vi "Acquisition Message Loop.vi"(6 "Acquisition Status Notifier":refnum<notifier>, 8 "error in (no error)":errorcluster, 9 "Data Queue":refnum<queue>, 10 "Data Notifier":refnum<notifier>, 11 "Message Queues":T1) -> (0 "error out":errorcluster)   [LabVIEW 2021, in "Acquisition.lvlib"]
doc: "Message loop for handling messages pertaining to the acquisition of data from the hardware."
uses:
  Acquisition.lvlib
  support/Message Queue/All Message Queues.ctl
  support/Message Queue/Message Cluster.ctl
  Acquired Data.ctl
  controls/Acquisition Status.ctl
  Acquisition State.ctl
  support/Message Queue/Enqueue Message (Single).vi
  <vilib>/Utility/error.llb/Error Cluster From Error Code.vi
  <vilib>/ErrorRing/Error Ring.xnode
  support/Message Queue/Message Queue.lvlib
panel:
  out "msgctr":i32
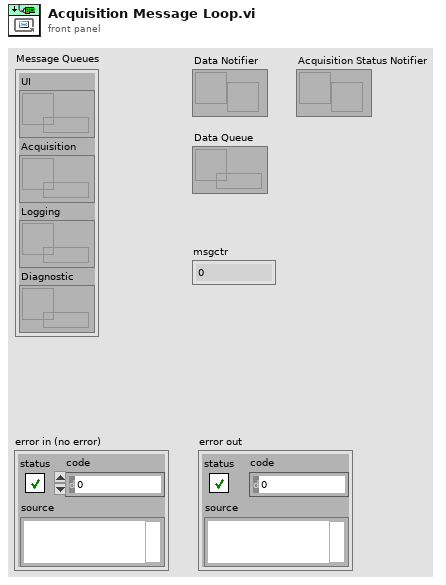
[diagram p1: front panel]
types:
  T1 = typedef "Message Queue.lvlib/All Message Queues.ctl" = cluster{"UI":refnum<queue>, "Acquisition":refnum<queue>, "Logging":refnum<queue>, "Diagnostic":refnum<queue>}
  T2 = typedef "Acquisition.lvlib/Acquisition State.ctl" = enum16{"Idle", "Acquiring"}
  T3 = typedef "Acquisition.lvlib/Host Resources.ctl" = cluster{"NI Software":T4[], "IO Devices":T5[]}
  T4 = typedef "Acquisition.lvlib/Host Software Package.ctl" = cluster{"ID":string, "Version":string}
  T5 = typedef "Acquisition.lvlib/Host IO Resource.ctl" = cluster{"Model Number":u32, "Alias":string, "Product Name":string, "Is Device":bool, "Is Chassis":bool, "Is Simulated":bool, "Slot":i32}
  T6 = typedef "Acquisition.lvlib/Hardware Configuration.ctl" = cluster{"Channel Settings":T7[], "Sensor Intervals":T10[], "Sensor Token":T12, "IO Context":T13}
  T7 = typedef "Acquisition.lvlib/Channel Settings.ctl" = cluster{"Name":string, "Terminal Information":cluster{"IO Device":T8, "Channel":i32, "Sensor Type":T9}, "Calibration Information":cluster{"Excitation Voltage":dbl, "Calibration Factor":dbl, "Zero Value":dbl, "Calibration Formula":string, "Units":string}}
  T8 = typedef "Acquisition.lvlib/IO Device.ctl" = enum16{"none", "9219", "9401"}
  T9 = typedef "Acquisition.lvlib/Sensor Type.ctl" = enum16{"Voltage", "Load", "Pressure", "Encoder"}
  T10 = typedef "Interval Timer.lvlib/Repeat Interval.ctl" = cluster{"Interval":T11, "Count":i32}
  T11 = typedef "Interval Timer.lvlib/Interval Length.ctl" = enum16{"Manual control", "1 second", "10 seconds", "30 seconds", "60 seconds", "600 seconds", "1200 seconds", "3600 seconds"}
  T12 = typedef "Interval Timer.lvlib/Interval Token.ctl" = cluster{"Next reading in ms":u32, "Interval Index":i32, "Interval Occurrence":i32}
  T13 = typedef "Acquisition.lvlib/IO Context.ctl" = cluster{"API":T14, "API Wire":variant}
  T14 = typedef "Acquisition.lvlib/IO API.ctl" = enum16{"Simulated", "DAQmx"}
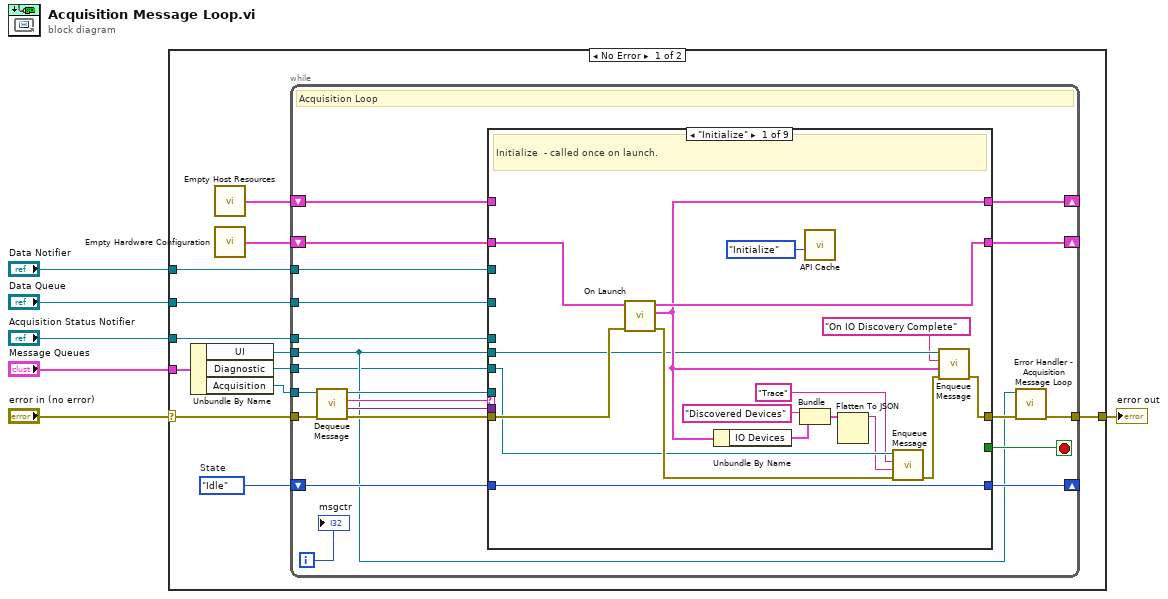
[diagram p0: block diagram]
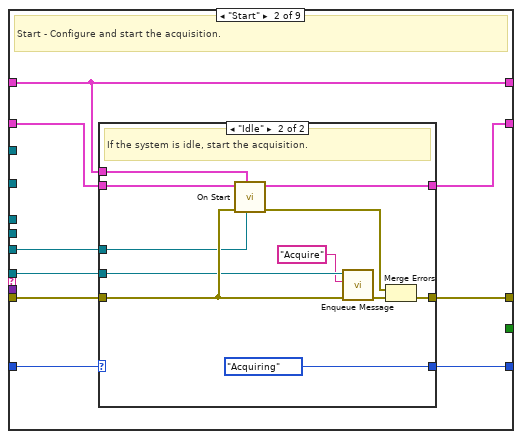
[diagram p2: hidden frame]
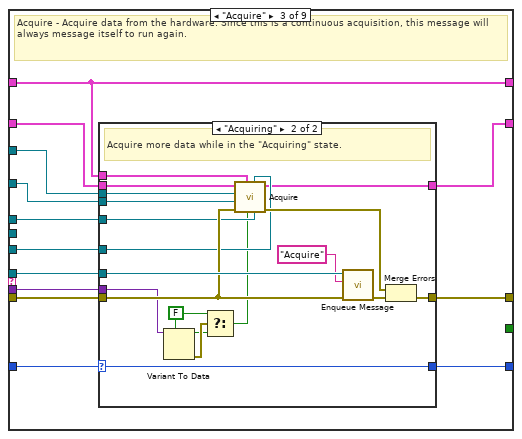
[diagram p4: hidden frame]
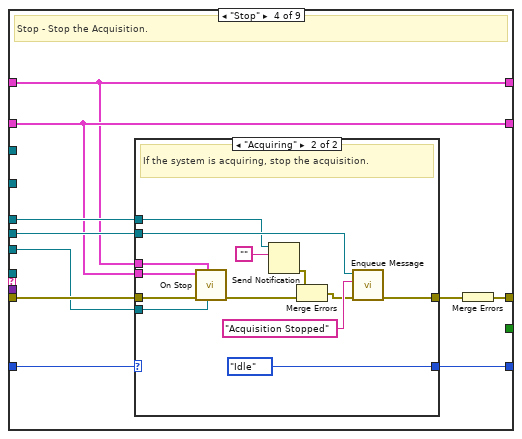
[diagram p6: hidden frame]
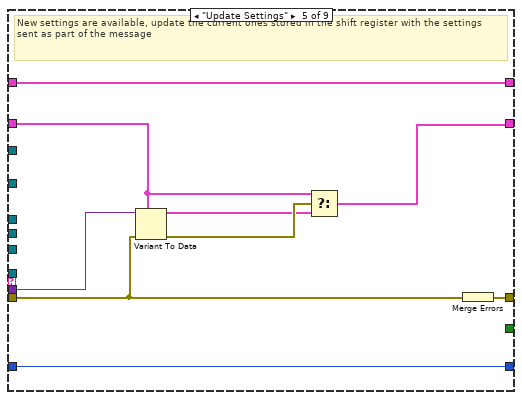
[diagram p8: hidden frame]
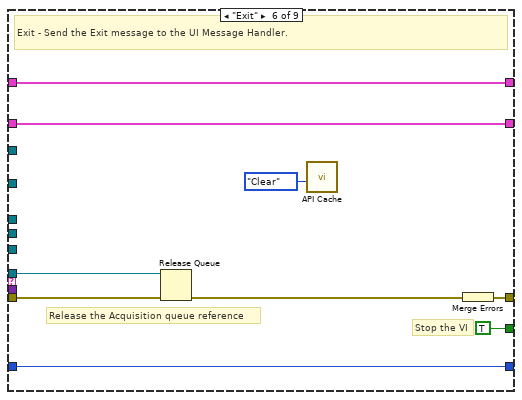
[diagram p9: hidden frame]
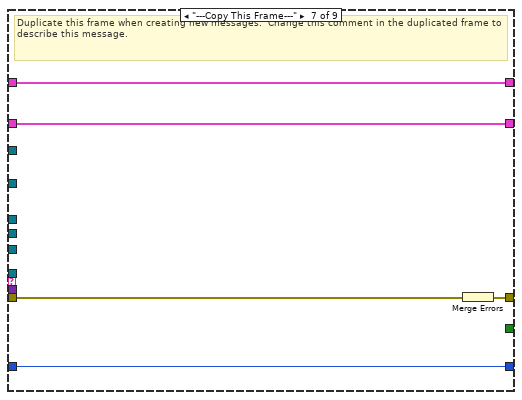
[diagram p10: hidden frame]
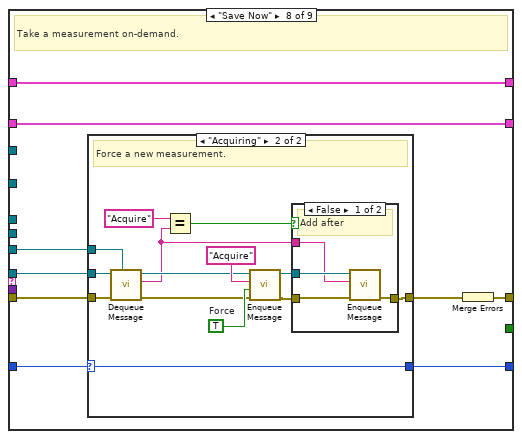
[diagram p11: hidden frame]
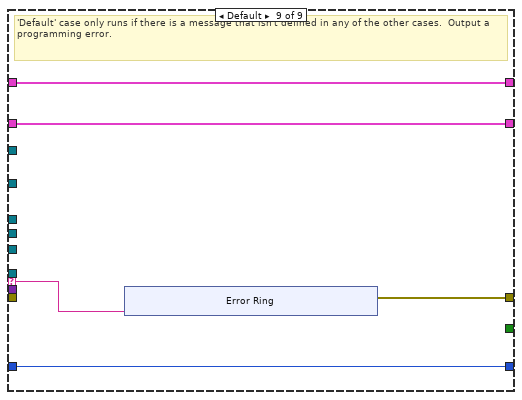
[diagram p14: hidden frame]
diagram:
  n1 = case shown="No Error" "error in (no error)" {
    selector: "error in (no error)" -> [w15 w205]
    tunnel: "Message Queues" -> [w18 _]
    tunnel: [w16 w205] -> w5
    tunnel: "Data Notifier" -> [w13 _]
    tunnel: "Data Queue" -> [w12 _]
    tunnel: "Acquisition Status Notifier" -> [w9 _]
    frame No Error {
      w11 = Acquisition_State."Idle"  # State
      n2 = Unbundle By Name(w18) -> ("UI"=w14:refnum<queue>, "Diagnostic"=w10:refnum<queue>, "Acquisition"=w17:refnum<queue>)
      n3 = call "Empty Host Resources.vi"() -> ("Host Resources"=w7:T3)
      n4 = call "Empty Hardware Configuration.vi"() -> ("Hardware Configuration"=w8:T6)
      n5 = while {
        tunnel: w17 -> [w32]
        shift-right: [w38] -> _
        shift-left: w8 -> [w39]
        tunnel: w14 -> [w24]
        tunnel: w13 -> [w31]
        tunnel: w12 -> [w30]
        shift-right: [w28] -> _
        shift-left: w11 -> [w29]
        tunnel: w15 -> [w36]
        tunnel: [w27] -> w16
        tunnel: w10 -> [w22]
        tunnel: w9 -> [w21]
        shift-right: [w19] -> _
        shift-left: w7 -> [w20]
        i -> [w23]
        stop <- w37 stop-if-true
        # "Acquisition Loop"
        n6 = call "Dequeue Message.vi"("error in (no error)"=w36, "Message Queue"=w32) -> ("error out"=w35:errorcluster, "Message Data"=w33:variant, "Message"=w34:string, "dup Message Queue"=w25:refnum<queue>)  [unwired: 6 in]
        n7 = case "Message Cases" shown="\"Initialize\"" w34 {
          selector: w34 -> [_ _ _ _ _ _ _ _ w194]
          tunnel: w25 -> [_ w63 w91 _ _ w152 _ w166 _]
          tunnel: w35 -> [w53 w64 w90 w123 w144 w154 w162 w168 _]
          tunnel: [w52 w65 w92 w124 w148 w156 w160 w171 w195] -> w26
          tunnel: w39 -> [w55 w60 w83 w117 w141 w155 w161 w165 w197]
          tunnel: [w54 w59 w82 w117 w140 w155 w161 w165 w197] -> w38
          tunnel: [_ _ _ _ _ TRUE _ _ _] -> w37
          tunnel: w33 -> [_ _ w85 _ w147 _ _ _ _]
          tunnel: w24 -> [w47 _ _ w119 _ _ _ _ _]
          tunnel: w31 -> [_ _ w89 _ _ _ _ _ _]
          tunnel: w30 -> [_ _ w88 _ _ _ _ _ _]
          tunnel: w29 -> [w56 w61 w86 w121 w143 w151 w159 w170 w196]
          tunnel: [w56 w62 w87 w120 w143 w151 w159 w169 w196] -> w28
          tunnel: w22 -> [w48 w57 w81 w116 _ _ _ w164 _]
          tunnel: w21 -> [_ _ w84 w118 _ _ _ _ _]
          tunnel: w20 -> [_ w58 w80 w115 w142 w150 w158 w163 w193]
          tunnel: [w51 w58 w80 w115 w142 w150 w158 w163 w193] -> w19
          frame "Initialize" {
            # "Initialize  - called once on launch."
            n8 = call "On Launch.vi"("error in (no error)"=w53, "Hardware Resources in"=w55) -> ("error out"=w50:errorcluster, "Host Resources"=w51:T3, "Hardware Resources out"=w54:T6)  [unwired: 7 in]
            n9 = Unbundle By Name(w51) -> ("IO Devices"=w44:T5[])
            n10 = Bundle("Message"="Discovered Devices", "IO Devices"=w44) -> (w42:cluster{"Message":string, "IO Devices":T5[]})  [unwired: 1 in]
            n11 = call "API Cache.vi"("Action"=enum16{"Initialize", "Get or Open", "Clear"}."Initialize") -> ()  [unwired: 9 in, 2 out]
            n12 = Flatten To JSON(anything=w42) -> (JSON string=w41:string)  [unwired: 2 in, 1 out]
            n13 = call-poly "Enqueue Message.vi"("error in (no error)"=w50, "Message Data"=w41, "Message"="Trace", "Message Queue"=w48) -> ("error out"=w49:errorcluster)  [unwired: 6 in, 1 out]
            n14 = call-poly "Enqueue Message.vi"("error in (no error)"=w49, "Message Data"=w51, "Message"="On IO Discovery Complete", "Message Queue"=w47) -> ("error out"=w52:errorcluster)  [unwired: 6 in, 1 out]
          }
          frame "Start" {
            # "Start - Configure and start the acquisition."
            n15 = case shown="\"Idle\"" w61 {
              selector: w61 -> [w66 _]
              tunnel: [w67 w79] -> w65
              tunnel: w60 -> [w68 w78]
              tunnel: w64 -> [w67 w77]
              tunnel: w63 -> [_ w75]
              tunnel: [w68 w71] -> w59
              tunnel: [w66 Acquisition_State."Acquiring" ("Acquisition State")] -> w62
              tunnel: w58 -> [_ w70]
              tunnel: w57 -> [_ w69]
              frame "Acquiring" {
                # "The system is already acquiring. Ignore the \"Start\" message."
              }
              frame "Idle" {
                # "If the system is idle, start the acquisition."
                n16 = call "On Start.vi"("Diagnostics Queue"=w69, "Host Resources"=w70, "error in (no error)"=w77, "Hardware Configuration in"=w78) -> ("error out"=w72:errorcluster, "Hardware Configuration out"=w71:T6)  [unwired: 6 in]
                n17 = call-poly "Enqueue Message.vi"("error in (no error)"=w77, "Message"="Acquire", "Message Queue"=w75) -> ("error out"=w76:errorcluster)  [unwired: 7 in, 1 out]
                n18 = Merge Errors(w72, w76) -> (w79:errorcluster)
              }
            }
          }
          frame "Acquire" {
            # "Acquire - Acquire data from the hardware. Since this is a continuous acquisition, this message will always message itself to run again."
            n19 = case shown="\"Acquiring\"" w86 {
              selector: w86 -> [w93 w106]
              tunnel: [w94 w114] -> w92
              tunnel: w91 -> [_ w112]
              tunnel: w90 -> [w94 w105]
              tunnel: [w95 w97] -> w82
              tunnel: w83 -> [w95 w110]
              tunnel: w89 -> [_ w108]
              tunnel: w88 -> [_ w107]
              tunnel: [w93 w106] -> w87
              tunnel: w85 -> [_ w104]
              tunnel: w84 -> [_ w100]
              tunnel: w81 -> [_ w99]
              tunnel: w80 -> [_ w98]
              frame "Idle" {
                # "Ignore \"Acquire\" messages when the acquisition is idle."
              }
              frame "Acquiring" {
                w103 = FALSE
                # "Acquire more data while in the \"Acquiring\" state."
                n20 = Variant To Data(type=w103, Variant=w104) -> (data=w101:bool, error out=w102:errorcluster)  [unwired: 1 in]
                n21 = Select(t=w103, s=w102, f=w101) -> (s? t:f=w96:bool)
                n22 = call "Acquire.vi"("Acquisition Status Notifier"=w100, "Diagnostics Queue"=w99, "Force?"=w96, "Host Resources"=w98, "error in (no error)"=w105, "Data Queue"=w107, "Data Notifier"=w108, "Hardware Resources in"=w110) -> ("error out"=w111:errorcluster, "Hardware Resources out"=w97:T6)  [unwired: 2 in]
                n23 = call-poly "Enqueue Message.vi"("error in (no error)"=w105, "Message"="Acquire", "Message Queue"=w112) -> ("error out"=w113:errorcluster)  [unwired: 7 in, 1 out]
                n24 = Merge Errors(w111, w113) -> (w114:errorcluster)
              }
            }
          }
          frame "Stop" {
            # "Stop - Stop the Acquisition."
            n25 = case shown="\"Acquiring\"" w121 {
              selector: w121 -> [w125 _]
              tunnel: w123 -> [w126 w139]
              tunnel: [w126 w135] -> w122
              tunnel: w117 -> [_ w137]
              tunnel: [w125 Acquisition_State."Idle" ("State")] -> w120
              tunnel: w119 -> [_ w134]
              tunnel: w118 -> [_ w130]
              tunnel: w116 -> [_ w128]
              tunnel: w115 -> [_ w127]
              frame "Idle" {
                # "The system is already idle. Ignore the \"Stop\" message."
              }
              frame "Acquiring" {
                # "If the system is acquiring, stop the acquisition."
                n26 = call "On Stop.vi"("Diagnostics Queue"=w128, "Host Resources"=w127, "error in (no error)"=w139, "Hardware Resources in"=w137) -> ("error out"=w138:errorcluster)  [unwired: 6 in, 1 out]
                n27 = Send Notification(notification="", notifier=w130) -> (error out=w131:errorcluster)  [unwired: 1 in, 1 out]
                n28 = Merge Errors(w131, w138) -> (w132:errorcluster)
                n29 = call-poly "Enqueue Message.vi"("error in (no error)"=w132, "Message"="Acquisition Stopped", "Message Queue"=w134) -> ("error out"=w135:errorcluster)  [unwired: 7 in, 1 out]
              }
            }
            n30 = Merge Errors(w122) -> (w124:errorcluster)
          }
          frame "Update Settings" {
            # "New settings are available, update the current ones stored in the shift register with the settings sent as part of the message"
            n31 = Variant To Data(error in=w144, type=w141, Variant=w147) -> (data=w145:T6, error out=w146:errorcluster)
            n32 = Select(t=w141, s=w146, f=w145) -> (s? t:f=w140:T6)
            n33 = Merge Errors(w144) -> (w148:errorcluster)
          }
          frame "Exit" {
            # "Release the Acquisition queue reference"
            # "Stop the VI"
            # "Exit - Send the Exit message to the UI Message Handler."
            n34 = Release Queue(queue=w152, error in (no error)=w154) -> (error out=w153:errorcluster)  [unwired: 1 in, 2 out]
            n35 = call "API Cache.vi"("Action"=enum16{"Initialize", "Get or Open", "Clear"}."Clear") -> ()  [unwired: 9 in, 2 out]
            n36 = Merge Errors(w153) -> (w156:errorcluster)
          }
          frame "---Copy This Frame---" {
            # "Duplicate this frame when creating new messages.  Change this comment in the duplicated frame to describe this message."
            n37 = Merge Errors(w162) -> (w160:errorcluster)
          }
          frame "Save Now" {
            # "Take a measurement on-demand."
            n38 = case shown="\"Acquiring\"" w170 {
              selector: w170 -> [w173 w187]
              tunnel: [w173 w187] -> w169
              tunnel: w168 -> [w172 w184]
              tunnel: [w172 w177] -> w167
              tunnel: w166 -> [_ w183]
              tunnel: w164 -> [_ w179]
              frame "Idle" {
                # "Ignore \"Save Now\" messages when idle."
              }
              frame "Acquiring" {
                w185 = TRUE  # Force
                # "Force a new measurement."
                n39 = call "Dequeue Message.vi"("Diagnostics Queue"=w179, "error in (no error)"=w184, "Message Queue"=w183) -> ("error out"=w181:errorcluster, "Message"=w174:string, "dup Message Queue"=w182:refnum<queue>)  [unwired: 5 in, 1 out]
                n40 = Equal?(x="Acquire" ("Message"), y=w174) -> (x = y?=w178:bool)
                n41 = call-poly "Enqueue Message.vi"("error in (no error)"=w181, "Message Data"=w185, "Message"="Acquire", "Message Queue"=w182) -> ("error out"=w176:errorcluster, "dup Message Queue"=w175:refnum<queue>)  [unwired: 6 in]
                n42 = case shown="False" w178 {
                  tunnel: [w191 w192] -> w177
                  tunnel: w176 -> [w190 w192]
                  tunnel: w175 -> [w189 _]
                  tunnel: w174 -> [w188 _]
                  frame False {
                    # "Add after"
                    n43 = call-poly "Enqueue Message.vi"("error in (no error)"=w190, "Message"=w188, "Message Queue"=w189) -> ("error out"=w191:errorcluster)  [unwired: 7 in, 1 out]
                  }
                  frame True {
                    # "Drop"
                  }
                }
              }
            }
            n44 = Merge Errors(w167) -> (w171:errorcluster)
          }
          frame Default {
            # "'Default' case only runs if there is a message that isn't defined in any of the other cases.  Output a programming error."
            n45 = xnode "Error Ring"("parameter 0"=w194) -> ("error out"=w195:errorcluster)
          }
        }
        n46 = call "Error Handler - Acquisition Message Loop.vi"("error in (no error)"=w26, "Message Queue"=w24) -> ("dup error in"=w27:errorcluster)  [unwired: 8 in, 1 out]
        "msgctr" <- w23
      }
    }
    frame Error {
    }
  }
  "error out" <- w5
